vi "Substitute Actor.vi"(10 "Substitute Actor in":refnum<class "Actor.lvclass">, 11 "Current Command Processor":refnum<class "Command Processor.lvclass">) -> (0 "error out":errorcluster, 2 "Substitute Actor out":refnum<class "Actor.lvclass">)   [LabVIEW 2013, in "Command Processor.lvlib" / "Command Processor.lvclass"]
doc: "(<B>Filename</B>: Actor Framework.lvlib:Actor.lvclass:Substitute Actor.vi)\n\nThis method copies information from the <b>Current Actor</b> to the <b>Substitute Actor</b>, including the to-self and the to-caller queue references. The purpose of this function is to allow an actor to define a method that replaces itself with another actor, useful for implementing a State Pattern Actor. Child classes should override this method to copy any additional fields that they need from the current to the substitute.\n\nThis method may return error code 678010: Illegal substitution. Overrides of this method may choose to return this error if the new actor is not one that is an appropriate substitute for the current actor, for whatever standards of \"appropriate\" are chosen for the current actor. If returning an error, override VIs should return the unmodified <b>Current Actor</b> as <b>Substitute Actor out</b>."
uses:
  Command Processor.lvclass
  <vilib>/ni/Actors/State Actor/State Actor/State Actor.lvclass
  <vilib>/ActorFramework/Actor/Actor.lvclass
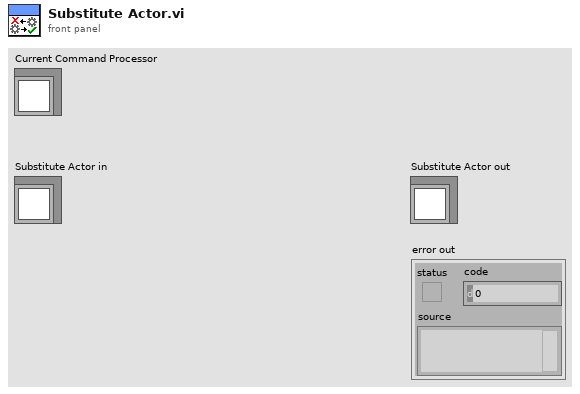
[diagram p1: front panel]
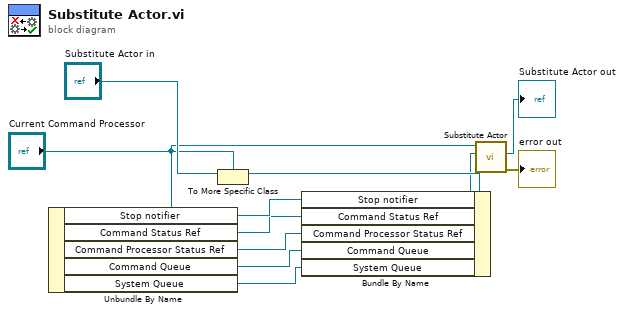
[diagram p0: block diagram]
diagram:
  n1 = Unbundle By Name("Current Command Processor") -> ("Stop notifier"=w5:refnum<notifier>, "Command Status Ref"=w4:refnum<vi>, "Command Processor Status Ref"=w3:refnum<vi>, "Command Queue"=w2:refnum<class "Message Enqueuer.lvclass">, "System Queue"=w1:refnum<class "Message Enqueuer.lvclass">)
  n2 = To More Specific Class(target class="Current Command Processor", reference="Substitute Actor in") -> (specific class reference=w7:refnum<class "Command Processor.lvclass">)  [unwired: 1 in, 1 out]
  n3 = Bundle By Name(cluster=w7, "Stop notifier"=w5, "Command Status Ref"=w4, "Command Processor Status Ref"=w3, "Command Queue"=w2, "System Queue"=w1) -> (w6:refnum<class "Command Processor.lvclass">)
  n4 = call-parent "Substitute Actor.vi"("Substitute Actor in"=w6, "Current Actor"="Current Command Processor") -> ("error out"=→"error out":errorcluster, "Substitute Actor out"=→"Substitute Actor out":refnum<class "Actor.lvclass">)  [unwired: 8 in]
